vi "Controls-Loop.vi"(7 "JSON cmd queue":refnum<queue>, 8 "error in":errorcluster, 9 "Control Data Notifier":refnum<notifier>, 11 "Message Queues":T1) -> (0 "error out":errorcluster)   [LabVIEW 2024]
uses:
  support/Message Queue/All Message Queues.ctl
  support/Message Queue/Message Cluster.ctl
  support/Control/Control Data Constant.ctl
  support/Control/StreamCluster_TypeDef.ctl
  <vilib>/ErrorRing/Error Ring.xnode
  support/Message Queue/Message Queue.lvlib
  Controls State.ctl
  support/Control/DAQmx Container.ctl
  Sequence/Sequence Structure.ctl
  support/Control/BBControl Parameters.ctl
  332b4253-326d-4d7b-9710-a01b345fab27.vi
  61c51413-b1d0-41cf-878e-839bc20d578b.vi
  c894b992-033a-4c8a-923e-e5ce24f73376.vi
  Globals.vi
  <vilib>/MediaMongrels Ltd/WebSockets/WebSockets/WebSocket Server/WebSocket Server.lvclass
  support/Control/wsControlStates.ctl
  <vilib>/JDP Science/JSONtext/JSONtext.lvlib
  a787d3b8-bd60-4c2f-a7c4-6a756d9c913a.vi
  81e338ed-8fff-406a-9241-f88d912df8f4.vi
  a40d114d-95b6-498c-b24b-cea1f821b3b0.vi
  f3c74be8-3d28-4f30-9817-3fb28c56d5a3.vi
panel:
  out "Loop-3 Iteration Clock (s) 2":dbl format="%10.8f"
  out "Loop-3 Iteration Counter 2":i32
  out "Loop-3 Iteration Counter":i32
  out "Loop-3 Iteration Clock (s)":dbl format="%10.8f"
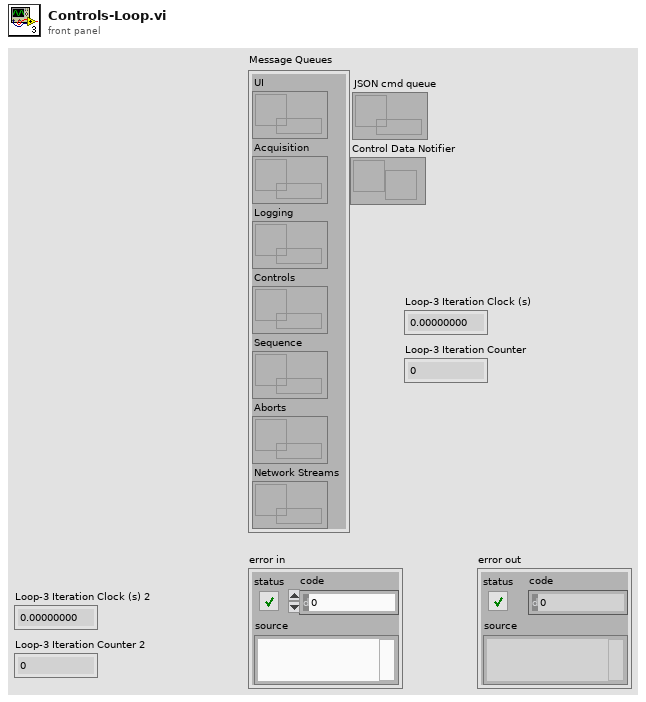
[diagram p1: front panel]
types:
  T1 = typedef "Message Queue.lvlib/All Message Queues.ctl" = cluster{"UI":refnum<queue>, "Acquisition":refnum<queue>, "Logging":refnum<queue>, "Controls":refnum<queue>, "Sequence":refnum<queue>, "Aborts":refnum<queue>, "Network Streams":refnum<queue>}
  T2 = typedef "wsControlStates.ctl" = enum16{"state_req", "state_update", "entrySequence", "control", "exitSequence"}
  T3 = cluster{"cmd set index":i32, "cmd subset index":i32, "cmd value":dbl, "t_ms":dbl, "refDes":string}
  T4 = typedef "Control Data Constant.ctl" = cluster{"Time (utc)":ext, "Data Out":cluster{"DO":bool[], "Module Number":string}[]}
  T5 = typedef "StreamCluster_TypeDef.ctl" = cluster{"DAQ":cluster{"ManagmentRate_Hz":i32, "StreamRate_Hz":i32, "StreamRate_ms":i32, "ManagmentRate_ms":i32, "refDesArray":cluster{"refDes-s":string[], "Module Number":string}[]}, "Modules":cluster{"Slot ID":i32, "Model Number":string, "Sample Rate s/S (Hz)":dbl, "Sensors":cluster{"refDes":string, "serialNumber":string, "modelNumber":string, "units":string, "balance":dbl, "sensitivity":dbl, "type":string, "inputTerminalConfiguration":string, "channelNumber":string, "taskName":string, "bridgeConfiguration":string, "excitationVoltage":dbl, "voltageExcitationSource":string, "nominalBridgeResistance":dbl, "firstElectricalValue":dbl, "secondElectricalValue":dbl, "firstPhysicalValue":dbl, "secondPhysicalValue":dbl, "electricalUnits":string}[]}[]}
  T6 = cluster{"refDes-s":string[], "Module Number":string}[]
  T7 = typedef "Controls State.ctl" = enum16{"Idle", "Control", "Sequencing", "Abort"}
  T8 = typedef "BBControl Parameters.ctl" = cluster{"Sequence Delay (s)":dbl, "Sequence Duration (s)":dbl, "BBControl Criteria":cluster{"Channel Name":i32, "Comparison":u16, "Set":dbl, "Enabled":bool, "Valve Name":i32, "Upper":dbl, "Lower":dbl}[]}
  T9 = typedef "DAQmx Container.ctl" = cluster{"DAQmx Analog In":refnum<k21>, "DAQmx Digital In":refnum<k21>, "DAQmx Digital Out":refnum<k21>, "DAQmx Analog Out":refnum<k21>, "DAQmx 6343":refnum<k21>, "DAQmx IG-Sense":refnum<k21>, "DAQmx Thermo":refnum<k21>, "DAQmx Bridge":refnum<k21>, "DAQmx Trigger":refnum<k21>}
  T10 = typedef "Sequence Structure.ctl" = cluster{"Sequence Controller":cluster{"Time (s)":dbl, "Enabled":bool, "Valve":u16[]}[], "Sequence Delay":dbl, "Sequence Duration":dbl}
  T11 = typedef "LVDateTimeRec.ctl" = cluster{"fractional second":dbl, "second":i32, "minute":i32, "hour":i32, "day of month":i32, "month":i32, "year":i32, "day of week":i32, "day of year":i32, "DST":i32}
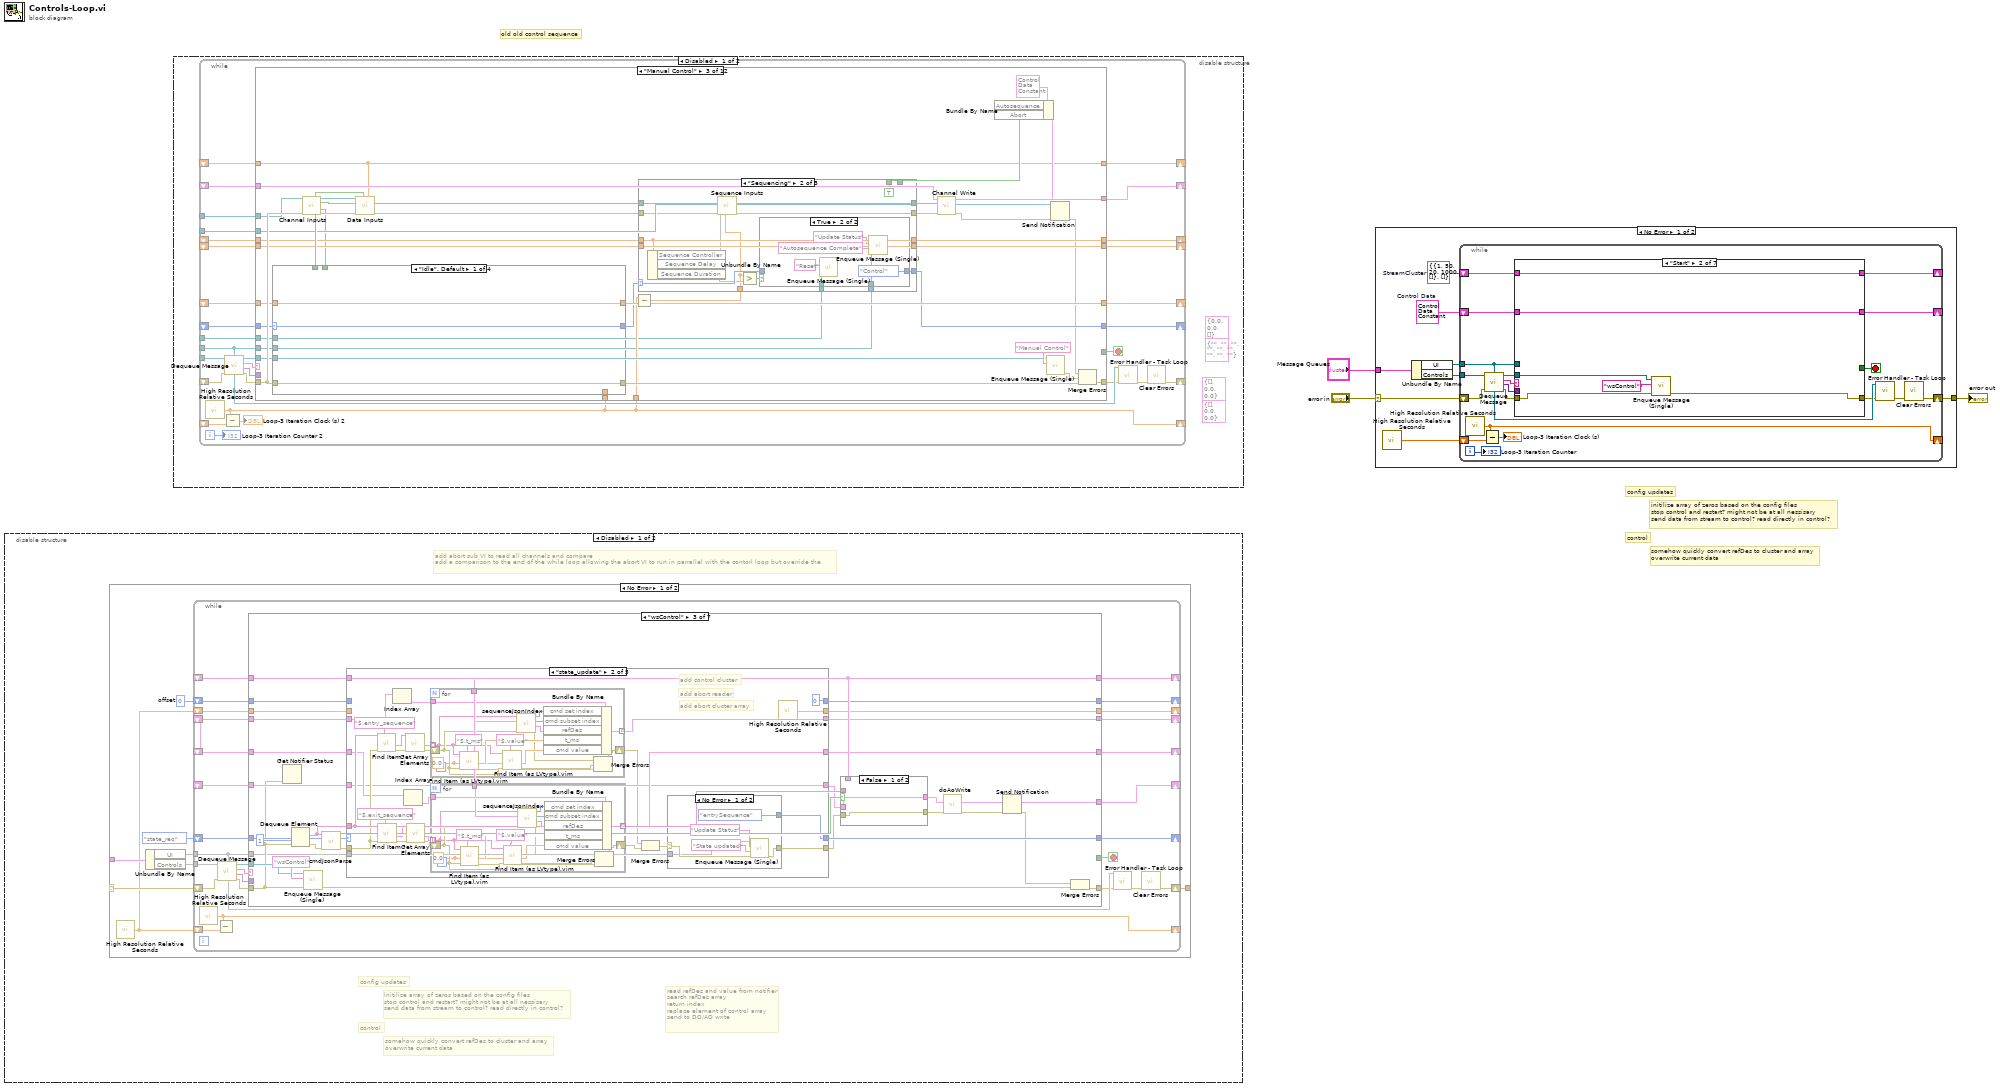
[diagram p0: block diagram]
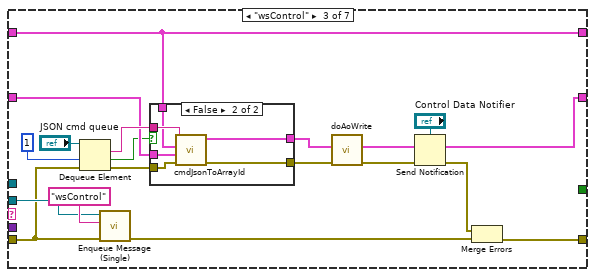
[diagram p3: hidden frame]
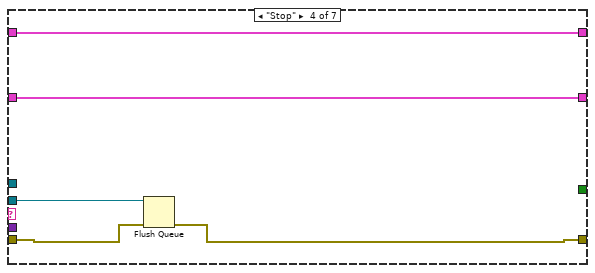
[diagram p5: hidden frame]
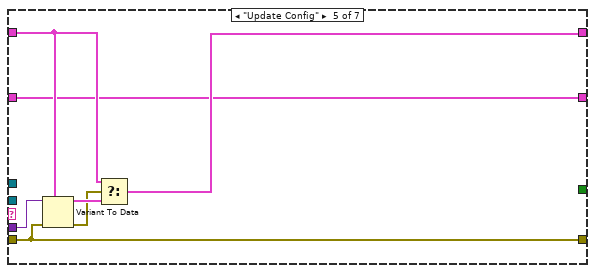
[diagram p6: hidden frame]
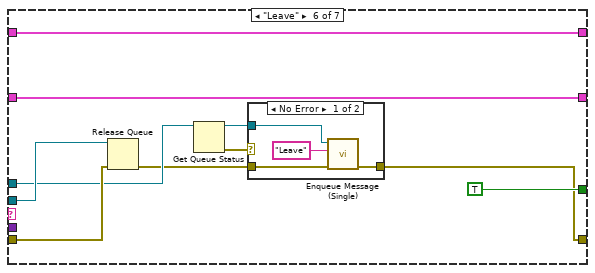
[diagram p7: hidden frame]
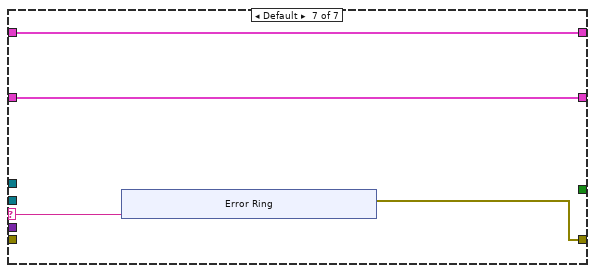
[diagram p9: hidden frame]
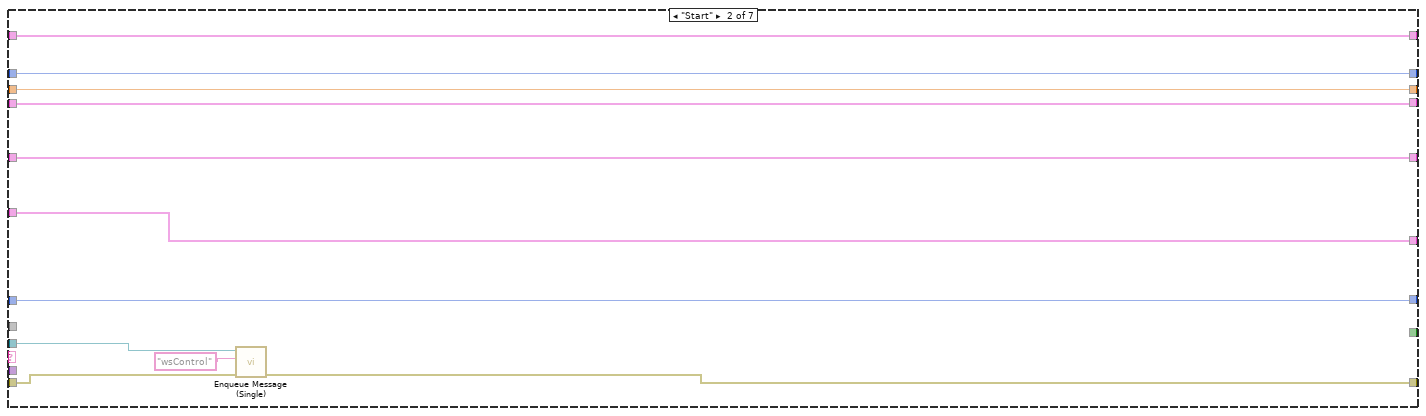
[diagram p12: hidden frame]
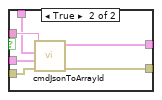
[diagram p13: hidden frame]
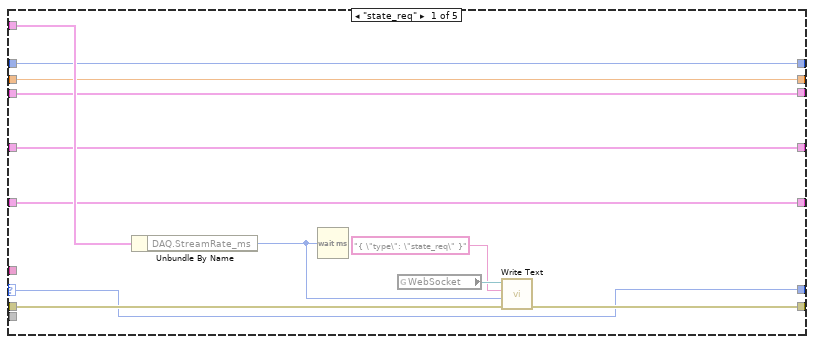
[diagram p14: hidden frame]
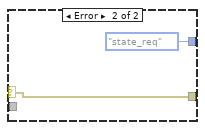
[diagram p15: hidden frame]
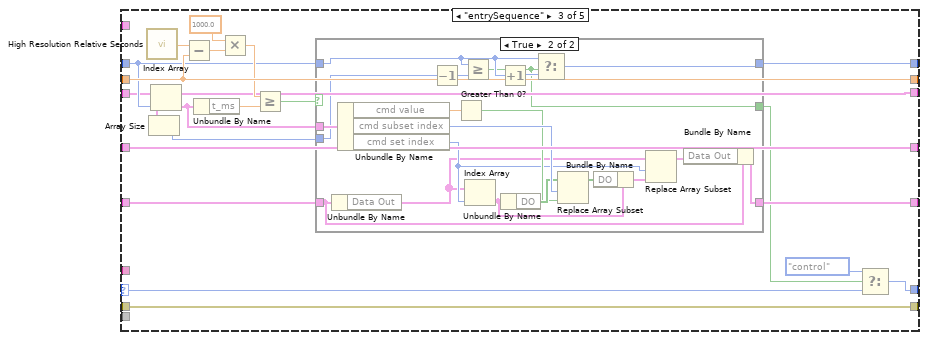
[diagram p16: hidden frame]
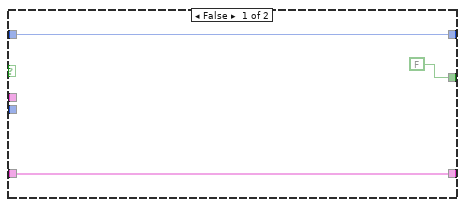
[diagram p17: hidden frame]
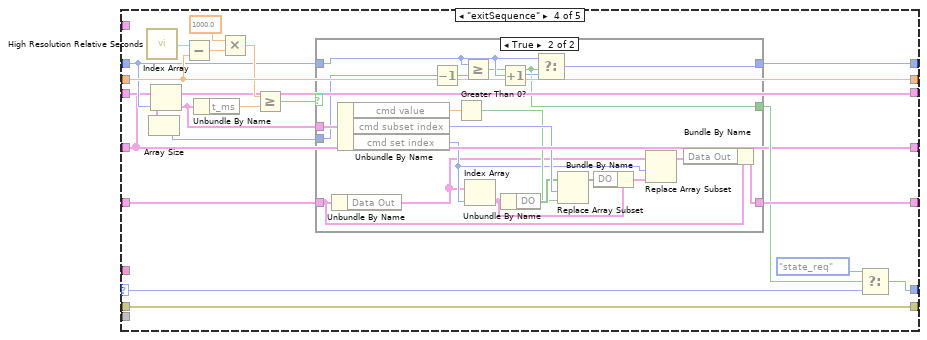
[diagram p18: hidden frame]
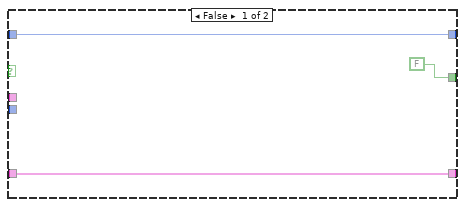
[diagram p19: hidden frame]
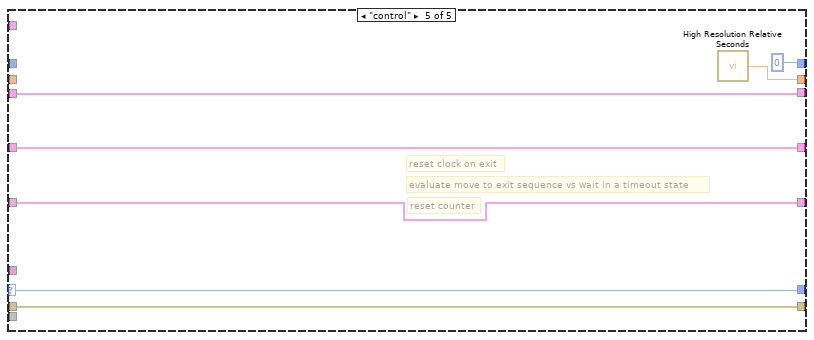
[diagram p20: hidden frame]
diagram:
  # "somehow quickly convert refDes to cluster and array\noverwrite current data"
  # "control"
  # "initilize array of zeros based on the config files \nstop control and restart? might not be at all nessisary\nsend data from stream to control? read directly in control?"
  # "config updates"
  # "old old control sequence"
  n1 = disable-structure shown="Disabled" {
    frame Disabled {
      # "add abort sub VI to read all channels and compare\nadd a comparison to the end of the while loop allowing the abort VI to run in parrallel with the contorl loop but override the"
      # "read refDes and value from notifier\nsearch refDes array\nreturn index\nreplace element of control array\nsend to DO/AO write"
      # "somehow quickly convert refDes to cluster and array\noverwrite current data"
      # "control"
      # "initilize array of zeros based on the config files \nstop control and restart? might not be at all nessisary\nsend data from stream to control? read directly in control?"
      # "config updates"
      n2 = case shown="No Error" w5 {
        selector: [w16 w347] -> w5
        tunnel: [w15 w347] -> _
        tunnel: [w14 _] -> w4
        frame No Error {
          w7 = 0  # offset
          n3 = call <vilib>:"High Resolution Relative Seconds.vi"() -> ("relative seconds"=w6:dbl)
          n4 = Unbundle By Name(w14) -> ("UI"=w13, "Controls"=w12)
          n5 = while {
            shift-right: [w32] -> w15
            shift-left: w16 -> [w42]
            tunnel: w13 -> [w36]
            tunnel: w12 -> [w43]
            shift-right: [w31] -> _
            shift-left: w6 -> [w35]
            shift-right: [w28] -> _
            shift-left: [w30] -> w11
            shift-right: [w27] -> _
            shift-left: [w29] -> w10
            shift-right: [w25] -> _
            shift-left: wsControlStates."state_req" -> [w26]
            shift-right: [w22] -> _
            shift-left: [w23] -> w8
            shift-right: [w21] -> _
            shift-left: w8 -> [w24]
            shift-right: [w17] -> _
            shift-left: w7 -> [w20]
            shift-right: [w18] -> _
            shift-left: w6 -> [w19]
            i -> [w34]
            stop <- w37 stop-if-true
            n6 = call <vilib>:"High Resolution Relative Seconds.vi"() -> ("relative seconds"=w31:dbl)
            n7 = Subtract(x=w31, y=w35) -> ()  [unwired: 1 out]
            n8 = call "Dequeue Message.vi"("error in (no error)"=w42, "Message Queue"=w43) -> ("error out"=w41:errorcluster, "Message Data"=w39:variant, "Message"=w38:string, "dup Message Queue"=w40:refnum<queue>)  [unwired: 6 in]
            n9 = case shown="\"wsControl\"" w38 {
              selector: w38 -> [_ _ _ _ _ _ w340]
              tunnel: [w52 w61 w94 w284 w302 w324 w341] -> w33
              tunnel: w41 -> [w52 w62 w77 w285 w302 w326 _]
              tunnel: w40 -> [_ w63 w92 w283 _ w327 _]
              tunnel: w39 -> [_ _ _ _ w303 _ _]
              tunnel: [_ _ _ _ _ TRUE _] -> w37
              tunnel: w36 -> [_ _ w71 _ _ w323 _]
              tunnel: w30 -> [w51 w60 w85 w282 w294 w318 w338]
              tunnel: w29 -> [w50 w59 w88 w281 w293 w319 w339]
              tunnel: [w51 w60 w82 w282 w292 w318 w338] -> w28
              tunnel: [w50 w59 w88 w281 w291 w319 w339] -> w27
              tunnel: w26 -> [w49 w57 w78 _ w290 w317 w337]
              tunnel: [w49 w57 w87 wsControlStates."state_req" ("controlStates") w290 w317 w337] -> w25
              tunnel: w24 -> [w48 w53 w73 w279 w286 w313 w333]
              tunnel: w23 -> [w47 w54 w72 w278 w287 w314 w334]
              tunnel: [w47 w54 w70 w278 w287 w314 w334] -> w22
              tunnel: [w48 w53 w69 w279 w286 w313 w333] -> w21
              tunnel: w20 -> [w45 w56 w67 w276 w289 w316 w336]
              tunnel: w19 -> [w46 w55 w66 w277 w288 w315 w335]
              tunnel: [w46 w55 w65 w277 w288 w315 w335] -> w18
              tunnel: [w45 w56 w64 w276 w289 w316 w336] -> w17
              frame "Initialize" {
              }
              frame "Start" {
                n10 = call "Enqueue Message (Single).vi"("error in (no error)"=w62, "Message"="wsControl", "Message Queue"=w63) -> ("error out"=w61:errorcluster)  [unwired: 7 in, 1 out]
              }
              frame "wsControl" {
                n11 = Get Notifier Status(error in (no error)=w77) -> ()  [unwired: 1 in, 5 out]
                n12 = Dequeue Element(timeout in ms (-1)=1, error in (no error)=w77) -> (element=w74:string, error out=w90:errorcluster)  [unwired: 1 in, 2 out]
                n13 = call "Enqueue Message (Single).vi"("error in (no error)"=w77, "Message"="wsControl", "Message Queue"=w92) -> ("error out"=w80:errorcluster)  [unwired: 7 in, 1 out]
                n14 = call "cmdJsonParse.vi"("error in"=w90, "controlStates"=w78, "cmdJson"=w74) -> ("error out"=w75:errorcluster, "controlStates"=w76:T2, "cmd"=w89:bool)  [unwired: 6 in]
                n15 = case shown="\"state_update\"" w76 {
                  selector: w76 -> [w105 _ w189 w232 w270]
                  tunnel: [w113 w117 w204 w246 w269] -> w84
                  tunnel: w75 -> [w112 w135 w204 w246 w269]
                  tunnel: w88 -> [w111 w125 _ _ _]
                  tunnel: [w105 w118 w186 w229 w270] -> w87
                  tunnel: w85 -> [w108 w123 w195 w238 w271]
                  tunnel: [w108 w123 w194 w237 w271] -> w68
                  tunnel: w74 -> [_ w136 _ _ _]
                  tunnel: w73 -> [w106 w126 w203 w227 w272]
                  tunnel: w72 -> [w107 w133 w185 w228 w273]
                  tunnel: w71 -> [_ w119 _ _ _]
                  tunnel: [w107 w131 w185 w228 w273] -> w70
                  tunnel: [w106 w124 w203 w227 w272] -> w69
                  tunnel: w67 -> [w104 _ w192 w235 _]
                  tunnel: w66 -> [w103 _ w201 w244 _]
                  tunnel: [w103 w116 w201 w244 w274] -> w65
                  tunnel: [w104 0 ("offset") w191 w234 0 ("offset")] -> w64
                  frame "state_req" {
                    n16 = Unbundle By Name(w111) -> ("DAQ.StreamRate_ms"=w109:i32)
                    n17 = Wait (ms)(milliseconds to wait=w109) -> ()  [unwired: 1 out]
                    n18 = global read "Globals.vi" "WebSocket"() -> (w114:refnum<class "WebSocket Server.lvclass">)
                    n19 = call-dynamic "Write Text.vi"("error in (no error)"=w112, "timeout ms (5000)"=w109, "String Data"="{ \"type\": \"state_req\" }", "WebSocket in"=w114) -> ("error out"=w113:errorcluster)  [unwired: 6 in, 1 out]
                  }
                  frame "state_update" {
                    # "add control cluster"
                    # "add abort cluster array"
                    # "add abort reader"
                    n20 = call <vilib>:"Find Item.vi"("$Path or Item Name"="$.entry_sequence", "error in (no error)"=w135, "JSON"=w136) -> ("error out"=w139:errorcluster, "<JSON>"=w138:string)  [unwired: 5 in, 2 out]
                    n21 = call <vilib>:"Find Item.vi"("$Path or Item Name"="$.exit_sequence", "error in (no error)"=w135, "JSON"=w136) -> ("error out"=w142:errorcluster, "<JSON>"=w141:string)  [unwired: 5 in, 2 out]
                    n22 = Index Array(array=w133) -> (element=w132:T3)  [unwired: 1 in]
                    n23 = Index Array(array=w126) -> (element=w127:T3)  [unwired: 1 in]
                    n24 = call <vilib>:"Get Array Elements.vi"("error in (no error)"=w139, "JSON"=w138) -> ("error out"=w130:errorcluster, "<JSON>"=w134:string[])  [unwired: 7 in, 1 out]
                    n25 = call <vilib>:"Get Array Elements.vi"("error in (no error)"=w142, "JSON"=w141) -> ("error out"=w128:errorcluster, "<JSON>"=w129:string[])  [unwired: 7 in, 1 out]
                    n26 = for {
                      tunnel: w134 -> [w172] mode=indexing
                      tunnel: w132 -> [w184]
                      tunnel: [w181] -> w131 mode=indexing
                      shift-right: [w168] -> w121
                      shift-left: w130 -> [w175]
                      tunnel: w125 -> [w180]
                      w174 = 0.0
                      n27 = call "Find Item (as LVtype).vim"("$Path or Item Name"="$.t_ms", "error in (no error)"=w175, "Data Type and Default Value"=w174, "JSON"=w172) -> ("error out"=w171:errorcluster, "Data"=w177:dbl)  [unwired: 4 in, 2 out]
                      n28 = call "Find Item (as LVtype).vim"("$Path or Item Name"="$.value", "error in (no error)"=w175, "Data Type and Default Value"=w174, "JSON"=w172) -> ("error out"=w170:errorcluster, "Data"=w173:dbl)  [unwired: 4 in, 2 out]
                      n29 = call "sequenceJsonIndex.vi"("error in"=w175, "StreamCluster"=w180, "JSON in"=w172) -> ("error out"=w169:errorcluster, "refDes"=w179:string, "cmd subset index"=w182:i32, "cmd set index"=w183:i32)  [unwired: 5 in]
                      n30 = Bundle By Name(cluster=w184, "cmd set index"=w183, "cmd subset index"=w182, "refDes"=w179, "t_ms"=w177, "cmd value"=w173) -> (w181:T3)
                      n31 = Merge Errors(w169, w170, w171) -> (w168:errorcluster)
                    }
                    n32 = for {
                      tunnel: w129 -> [w155] mode=indexing
                      tunnel: w127 -> [w167]
                      tunnel: [w164] -> w124 mode=indexing
                      shift-right: [w151] -> w122
                      shift-left: w128 -> [w158]
                      tunnel: w125 -> [w163]
                      w157 = 0.0
                      n33 = call "Find Item (as LVtype).vim"("$Path or Item Name"="$.t_ms", "error in (no error)"=w158, "Data Type and Default Value"=w157, "JSON"=w155) -> ("error out"=w154:errorcluster, "Data"=w160:dbl)  [unwired: 4 in, 2 out]
                      n34 = call "Find Item (as LVtype).vim"("$Path or Item Name"="$.value", "error in (no error)"=w158, "Data Type and Default Value"=w157, "JSON"=w155) -> ("error out"=w153:errorcluster, "Data"=w156:dbl)  [unwired: 4 in, 2 out]
                      n35 = call "sequenceJsonIndex.vi"("error in"=w158, "StreamCluster"=w163, "JSON in"=w155) -> ("error out"=w152:errorcluster, "refDes"=w162:string, "cmd subset index"=w165:i32, "cmd set index"=w166:i32)  [unwired: 5 in]
                      n36 = Bundle By Name(cluster=w167, "cmd set index"=w166, "cmd subset index"=w165, "refDes"=w162, "t_ms"=w160, "cmd value"=w156) -> (w164:T3)
                      n37 = Merge Errors(w152, w153, w154) -> (w151:errorcluster)
                    }
                    n38 = Merge Errors(w121, w122) -> (w120:errorcluster)
                    n39 = case shown="No Error" w120 {
                      selector: w120 -> [w147 w149]
                      tunnel: w119 -> [w145 _]
                      tunnel: [wsControlStates."entrySequence" wsControlStates."state_req"] -> w118
                      tunnel: [w143 w149] -> w117
                      frame No Error {
                        n40 = call "Enqueue Message (Single).vi"("error in (no error)"=w147, "Message Data"="State updated", "Message"="Update Status", "Message Queue"=w145) -> ("error out"=w143:errorcluster)  [unwired: 6 in, 1 out]
                      }
                      frame Error {
                      }
                    }
                    n41 = call <vilib>:"High Resolution Relative Seconds.vi"() -> ("relative seconds"=w116:dbl)
                  }
                  frame "entrySequence" {
                    n42 = call <vilib>:"High Resolution Relative Seconds.vi"() -> ("relative seconds"=w202:dbl)
                    n43 = Array Size(array=w185) -> (size(s)=w190:i32)
                    n44 = Index Array(array=w185, index=w192) -> (element=w193:T3)
                    n45 = Subtract(x=w202, y=w201) -> (x-y=w200:dbl)
                    n46 = Unbundle By Name(w193) -> ("t_ms"=w198:dbl)
                    n47 = Multiply(x=1000.0, y=w200) -> (x*y=w197:dbl)
                    n48 = Greater Or Equal?(x=w197, y=w198) -> (x >= y?=w196:bool)
                    n49 = case shown="True" w196 {
                      tunnel: w195 -> [w207 w212]
                      tunnel: [w207 w211] -> w194
                      tunnel: w193 -> [_ w223]
                      tunnel: w192 -> [w206 w224]
                      tunnel: [w206 w225] -> w191
                      tunnel: w190 -> [_ w209]
                      tunnel: [FALSE w210] -> w188
                      frame False {
                      }
                      frame True {
                        n50 = Unbundle By Name(w212) -> ("Data Out"=w214:cluster{"DO":bool[], "Module Number":string}[])
                        n51 = Unbundle By Name(w223) -> ("cmd value"=w222:dbl, "cmd subset index"=w221:i32, "cmd set index"=w215:i32)
                        n52 = Decrement(x=w209) -> (x-1=w208:i32)
                        n53 = Greater Than 0?(x=w222) -> (x > 0?=w219:bool)
                        n54 = Greater Or Equal?(x=w224, y=w208) -> (x >= y?=w210:bool)
                        n55 = Index Array(array=w214, index=w215) -> (element=w218:cluster{"DO":bool[], "Module Number":string})
                        n56 = Increment(x=w224) -> (x+1=w226:i32)
                        n57 = Unbundle By Name(w218) -> ("DO"=w220:bool[])
                        n58 = Select(t=w224, s=w210, f=w226) -> (s? t:f=w225:i32)
                        n59 = Replace Array Subset(array=w220, new element=w219, index=w221) -> (w217:bool[])
                        n60 = Bundle By Name(cluster=w218, "DO"=w217) -> (w216:cluster{"DO":bool[], "Module Number":string})
                        n61 = Replace Array Subset(array=w214, new element=w216, index=w215) -> (w213:cluster{"DO":bool[], "Module Number":string}[])
                        n62 = Bundle By Name(cluster=w212, "Data Out"=w213) -> (w211:T4)
                      }
                    }
                    n63 = Select(t=wsControlStates."control", s=w188, f=w189) -> (s? t:f=w186:T2)
                  }
                  frame "exitSequence" {
                    n64 = call <vilib>:"High Resolution Relative Seconds.vi"() -> ("relative seconds"=w245:dbl)
                    n65 = Array Size(array=w227) -> (size(s)=w233:i32)
                    n66 = Index Array(array=w227, index=w235) -> (element=w236:T3)
                    n67 = Subtract(x=w245, y=w244) -> (x-y=w243:dbl)
                    n68 = Unbundle By Name(w236) -> ("t_ms"=w241:dbl)
                    n69 = Multiply(x=1000.0, y=w243) -> (x*y=w240:dbl)
                    n70 = Greater Or Equal?(x=w240, y=w241) -> (x >= y?=w239:bool)
                    n71 = case shown="True" w239 {
                      tunnel: w238 -> [w249 w254]
                      tunnel: [w249 w253] -> w237
                      tunnel: w236 -> [_ w265]
                      tunnel: w235 -> [w248 w266]
                      tunnel: [w248 w267] -> w234
                      tunnel: w233 -> [_ w251]
                      tunnel: [FALSE w252] -> w231
                      frame False {
                      }
                      frame True {
                        n72 = Unbundle By Name(w254) -> ("Data Out"=w256:cluster{"DO":bool[], "Module Number":string}[])
                        n73 = Unbundle By Name(w265) -> ("cmd value"=w264:dbl, "cmd subset index"=w263:i32, "cmd set index"=w257:i32)
                        n74 = Decrement(x=w251) -> (x-1=w250:i32)
                        n75 = Greater Than 0?(x=w264) -> (x > 0?=w261:bool)
                        n76 = Greater Or Equal?(x=w266, y=w250) -> (x >= y?=w252:bool)
                        n77 = Index Array(array=w256, index=w257) -> (element=w260:cluster{"DO":bool[], "Module Number":string})
                        n78 = Increment(x=w266) -> (x+1=w268:i32)
                        n79 = Unbundle By Name(w260) -> ("DO"=w262:bool[])
                        n80 = Select(t=w266, s=w252, f=w268) -> (s? t:f=w267:i32)
                        n81 = Replace Array Subset(array=w262, new element=w261, index=w263) -> (w259:bool[])
                        n82 = Bundle By Name(cluster=w260, "DO"=w259) -> (w258:cluster{"DO":bool[], "Module Number":string})
                        n83 = Replace Array Subset(array=w256, new element=w258, index=w257) -> (w255:cluster{"DO":bool[], "Module Number":string}[])
                        n84 = Bundle By Name(cluster=w254, "Data Out"=w255) -> (w253:T4)
                      }
                    }
                    n85 = Select(t=wsControlStates."state_req", s=w231, f=w232) -> (s? t:f=w229:T2)
                  }
                  frame "control" {
                    # "reset counter"
                    # "evaluate move to exit sequence vs wait in a timeout state"
                    # "reset clock on exit"
                    n86 = call <vilib>:"High Resolution Relative Seconds.vi"() -> ("relative seconds"=w274:dbl)
                  }
                }
                n87 = case shown="False" w89 {
                  tunnel: [w95 w102] -> w86
                  tunnel: w74 -> [_ w101]
                  tunnel: w88 -> [_ w100]
                  tunnel: w68 -> [w96 w99]
                  tunnel: [w96 w98] -> w83
                  tunnel: w84 -> [w95 w97]
                  frame False {
                  }
                  frame True {
                    n88 = call "cmdJsonToArrayId.vi"("error in"=w97, "Control Data"=w99, "StreamCluster"=w100, "JSON in"=w101) -> ("error out"=w102:errorcluster, "Control Data"=w98:T4)  [unwired: 6 in]
                  }
                }
                n89 = call "doAoWrite.vi"("error in"=w86, "Control Data"=w83) -> ("error out"=w91:errorcluster, "Control Data"=w82:T4)  [unwired: 7 in, 1 out]
                n90 = Send Notification(notification=w82, error in (no error)=w91) -> (error out=w81:errorcluster)  [unwired: 1 in, 1 out]
                n91 = Merge Errors(w81, w80) -> (w94:errorcluster)
              }
              frame "Stop" {
                n92 = Flush Queue(queue=w283, error in (no error)=w285) -> (error out=w284:errorcluster)  [unwired: 2 out]
              }
              frame "Update Config" {
                n93 = Variant To Data(error in=w302, type=w293, Variant=w303) -> (data=w304:T5, error out=w301:errorcluster)
                n94 = Select(t=w293, s=w301, f=w304) -> (s? t:f=w291:T5)
                n95 = Unbundle By Name(w291) -> ("DAQ.refDesArray"=w295:T6)
                n96 = Array Size(array=w295) -> (size(s)=w298:i32)
                n97 = Unbundle By Name(w294) -> ("Data Out"=w297:cluster{"DO":bool[], "Module Number":string}[])
                n98 = Index Array(array=w297) -> (element=w296:cluster{"DO":bool[], "Module Number":string})  [unwired: 1 in]
                n99 = for {
                  N: w298 -> [_]
                  tunnel: w295 -> [w307] mode=indexing
                  tunnel: w296 -> [w310]
                  tunnel: [w308] -> w300 mode=indexing
                  n100 = Unbundle(w307) -> ("refDes-s"=w306:string[], "Module Number"=w305:string)
                  n101 = Array Size(array=w306) -> (size(s)=w311:i32)
                  n102 = Initialize Array(FALSE, w311) -> (w309:bool[])
                  n103 = Bundle By Name(cluster=w310, "DO"=w309, "Module Number"=w305) -> (w308:cluster{"DO":bool[], "Module Number":string})
                }
                n104 = Bundle By Name(cluster=w294, "Data Out"=w300) -> (w299:T4)
                n105 = Select(t=w294, s=w301, f=w299) -> (s? t:f=w292:T4)
              }
              frame "Leave" {
                n106 = Release Queue(queue=w327, error in (no error)=w326) -> (error out=w321:errorcluster)  [unwired: 1 in, 2 out]
                n107 = Get Queue Status(queue=w323) -> (queue out=w322:refnum<queue>, error out=w320:errorcluster)  [unwired: 2 in, 6 out]
                n108 = case shown="No Error" w320 {
                  tunnel: [w330 w332] -> w324
                  tunnel: w322 -> [w329 _]
                  tunnel: w321 -> [w328 w332]
                  frame No Error {
                    n109 = call "Enqueue Message (Single).vi"("error in (no error)"=w328, "Message"="Leave", "Message Queue"=w329) -> ("error out"=w330:errorcluster)  [unwired: 7 in, 1 out]
                  }
                  frame Error {
                  }
                }
              }
              frame Default {
                n110 = xnode "Error Ring"("parameter 0"=w340) -> ("error out"=w341:errorcluster)
              }
            }
            n111 = call "Error Handler - Task Loop.vi"("error in (no error)"=w33, "Message Queue"=w36) -> ("dup error in"=w44:errorcluster)  [unwired: 8 in, 1 out]
            n112 = call <vilib>:"Clear Errors.vi"("error in (no error)"=w44) -> ("error out"=w32:errorcluster)  [unwired: 5 in, 1 out]
          }
        }
        frame Error {
        }
      }
    }
    frame Enabled {
    }
  }
  n113 = disable-structure shown="Disabled" {
    frame Disabled {
      (unwired) T8 {"Sequence Delay (s)"=0.0, "Sequence Duration (s)"=0.0, "BBControl Criteria"=[]} ("BBControl Parameters")
      (unwired) T9 {"DAQmx Analog In"="", "DAQmx Digital In"="", "DAQmx Digital Out"="", "DAQmx Analog Out"="", "DAQmx 6343"="", "DAQmx IG-Sense"="", "DAQmx Thermo"="", "DAQmx Bridge"="", "DAQmx Trigger"=""} ("DAQmx Container")
      (unwired) T10 {"Sequence Controller"=[], "Sequence Delay"=0.0, "Sequence Duration"=0.0} ("Sequence Conditions")
      (unwired) T10 {"Sequence Controller"=[], "Sequence Delay"=0.0, "Sequence Duration"=0.0} ("Sequence Conditions")
      n114 = while {
        shift-right: [w350] -> _
        shift-left: _ -> [w375]
        tunnel: _ -> [w367]
        tunnel: _ -> [w376]
        shift-right: [w369] -> _
        shift-left: _ -> [w370]
        shift-right: [w357] -> _
        shift-left: _ -> [w365]
        tunnel: _ -> [w362]
        shift-right: [w360] -> _
        shift-left: _ -> [w361]
        tunnel: _ -> [w359]
        tunnel: _ -> [w358]
        shift-right: [w356] -> _
        shift-left: _ -> [w355]
        shift-right: [w353] -> _
        shift-left: _ -> [w354]
        shift-right: [w351] -> _
        shift-left: _ -> [w352]
        shift-right: [w348] -> _
        shift-left: _ -> [w349]
        i -> [w364]
        stop <- w368 stop-if-true
        n115 = call <vilib>:"High Resolution Relative Seconds.vi"() -> ("relative seconds"=w357:dbl)
        n116 = Subtract(x=w357, y=w365) -> (x-y=→"Loop-3 Iteration Clock (s) 2":dbl)
        n117 = call "Dequeue Message.vi"("error in (no error)"=w375, "Message Queue"=w376) -> ("error out"=w374:errorcluster, "Message Data"=w372:variant, "Message"=w371:string, "dup Message Queue"=w373:refnum<queue>)  [unwired: 6 in]
        n118 = case shown="\"Manual Control\"" w371 {
          selector: w371 -> [_ _ _ _ _ _ _ _ _ _ _ w686]
          tunnel: [w384 w390 w439 w590 w597 w604 w620 w630 w643 w654 w670 w687] -> w363
          tunnel: w374 -> [w384 w391 w442 w570 w597 w605 w622 w630 w643 w654 w673 _]
          tunnel: w373 -> [_ w392 w434 w586 _ w603 w621 _ _ _ w674 _]
          tunnel: w372 -> [_ _ _ _ _ _ w624 w636 w647 w658 _ _]
          tunnel: w370 -> [w383 w394 w440 w574 _ w607 w623 w635 w646 w657 w671 w685]
          tunnel: [w383 w393 w418 w574 Controls_State."Abort" ("Controls State") w606 w623 w635 w646 w657 w671 w685] -> w369
          tunnel: [w382 w389 w438 w589 w593 w602 w625 w631 w644 w655 w665 w684] -> w360
          tunnel: [_ _ _ _ _ _ _ _ _ _ TRUE _] -> w368
          tunnel: w367 -> [_ _ w413 _ _ _ _ _ _ _ w669 _]
          tunnel: w362 -> [_ _ w436 _ _ _ _ _ _ _ _ _]
          tunnel: w361 -> [w382 w389 w437 w588 w593 w602 w618 w631 w644 w655 w665 w684]
          tunnel: w359 -> [_ _ w406 _ _ _ _ _ _ _ _ _]
          tunnel: w358 -> [_ _ w410 w582 _ _ _ _ _ _ _ _]
          tunnel: w357 -> [_ _ w432 _ w594 _ _ _ _ _ _ _]
          tunnel: w357 -> [_ _ w429 _ _ _ _ _ _ _ _ _]
          tunnel: [w381 w388 w430 w573 w594 w601 w617 w634 w645 w656 w664 w683] -> w356
          tunnel: w355 -> [w381 w388 w431 w573 _ w601 w617 w634 w645 w656 w664 w683]
          tunnel: w354 -> [w380 w387 w416 w571 w595 w600 w616 w633 w640 w653 w663 w682]
          tunnel: [w380 w387 w415 w571 w595 w600 w616 w632 w640 w653 w663 w682] -> w353
          tunnel: w352 -> [w379 w386 w417 w572 w596 w599 w615 w629 w642 w652 w662 w681]
          tunnel: [w379 w386 w414 w572 w596 w599 w615 w629 w641 w652 w662 w681] -> w351
          tunnel: w349 -> [w378 w385 w402 w580 w591 w598 w614 w628 w639 w651 w661 w680]
          tunnel: [w378 w385 w402 w580 w591 w598 w614 w628 w639 w650 w661 w680] -> w348
          frame "Initialize" {
          }
          frame "Start" {
            n119 = case shown="\"Idle\", Default" w394 {
              selector: w394 -> [_ w401]
              tunnel: [Controls_State."Control" ("Controls State") w401] -> w393
              tunnel: w392 -> [w398 _]
              tunnel: w391 -> [w396 w400]
              tunnel: [w395 w400] -> w390
              frame "Idle", Default {
                n120 = call "Enqueue Message (Single).vi"("error in (no error)"=w396, "Message"="wsControl", "Message Queue"=w398) -> ("error out"=w395:errorcluster)  [unwired: 7 in, 1 out]
              }
              frame "Control" {
              }
            }
          }
          frame "Manual Control" {
            n121 = call "Channel Inputs.vi"("Data Notifier"=w436, "error in"=w442) -> ("BangBang\nArm out"=w403:bool, "Data Notifier out"=w426:refnum<notifier>, "Actuation Array"=w425:bool[], "Auto-sequence"=w407:bool, "Abort"=w428:bool, "error out"=w427:errorcluster)  [unwired: 8 in]
            n122 = case shown="\"Idle\", Default" w440 {
              selector: w440 -> [w492 w498 w525 w552]
              tunnel: w434 -> [_ w500 w527 w554]
              tunnel: w442 -> [w491 w499 w526 w553]
              tunnel: [w491 w503 w529 w557] -> w441
              tunnel: [w492 w504 w530 w558] -> w424
              tunnel: w413 -> [_ w501 w528 w555]
              tunnel: w406 -> [_ w502 w520 w556]
              tunnel: w407 -> [_ w494 _ w548]
              tunnel: w428 -> [_ _ w524 w545]
              tunnel: w432 -> [_ w497 w523 w551]
              tunnel: [w490 w496 w522 w550] -> w430
              tunnel: w431 -> [w490 w495 w521 w549]
              frame "Idle", Default {
              }
              frame "Control" {
                n123 = call "RisingEdgeDetector.vim"("Data"=w494) -> ("Edge?"=w493:bool)  [unwired: 4 in]
                n124 = case shown="True" w493 {
                  tunnel: [w507 Controls_State."Sequencing" ("Controls State")] -> w504
                  tunnel: w502 -> [_ w518]
                  tunnel: w499 -> [w506 w516]
                  tunnel: [w506 w513] -> w503
                  tunnel: w501 -> [_ w510]
                  tunnel: w500 -> [_ _]
                  tunnel: w498 -> [w507 _]
                  tunnel: [w505 w512] -> w496
                  tunnel: w497 -> [_ w512]
                  tunnel: w495 -> [w505 _]
                  frame False {
                  }
                  frame True {
                    n125 = call "Enqueue Message (Single).vi"("error in (no error)"=w516, "Message"="Start", "Message Queue"=w518) -> ("error out"=w508:errorcluster)  [unwired: 7 in, 1 out]
                    n126 = call "Enqueue Message (Single).vi"("error in (no error)"=w508, "Message"="Autosequence Start", "Message Queue"=w510) -> ("error out"=w509:errorcluster)  [unwired: 7 in, 1 out]
                    n127 = call "Enqueue Message (Single).vi"("error in (no error)"=w509, "Message Data"="Autosequence Started", "Message"="Update Status", "Message Queue"=w510) -> ("error out"=w513:errorcluster)  [unwired: 6 in, 1 out]
                  }
                }
              }
              frame "Sequencing" {
                n128 = case shown="True" w524 {
                  tunnel: [w533 Controls_State."Abort" ("Controls State")] -> w530
                  tunnel: w520 -> [_ w542]
                  tunnel: w526 -> [w532 w541]
                  tunnel: [w532 w537] -> w529
                  tunnel: w528 -> [_ w536]
                  tunnel: w527 -> [_ _]
                  tunnel: w525 -> [w533 _]
                  tunnel: w523 -> [_ w534]
                  tunnel: [w531 w534] -> w522
                  tunnel: w521 -> [w531 _]
                  frame False {
                  }
                  frame True {
                    n129 = call "Enqueue Message (Single).vi"("error in (no error)"=w541, "Message"="Reset", "Message Queue"=w542) -> ("error out"=w538:errorcluster)  [unwired: 7 in, 1 out]
                    n130 = call "Enqueue Message (Single).vi"("error in (no error)"=w538, "Message Data"="Manual Abort", "Message"="Update Status", "Message Queue"=w536) -> ("error out"=w537:errorcluster)  [unwired: 6 in, 1 out]
                  }
                }
              }
              frame "Abort" {
                n131 = call "FallingEdgeDetector.vim"("Data"=w545) -> ("Edge?"=w544:bool)  [unwired: 4 in]
                n132 = Not(x=w548) -> (.not. x?=w546:bool)
                n133 = And(x=w546, y=w544) -> (x .and. y?=w547:bool)
                n134 = case shown="True" w547 {
                  tunnel: [w561 Controls_State."Control" ("Controls State")] -> w558
                  tunnel: w556 -> [_ _]
                  tunnel: w553 -> [w560 w562]
                  tunnel: [w560 w565] -> w557
                  tunnel: w555 -> [_ w564]
                  tunnel: w554 -> [_ _]
                  tunnel: w552 -> [w561 _]
                  tunnel: w551 -> [_ w563]
                  tunnel: [w559 w563] -> w550
                  tunnel: w549 -> [w559 _]
                  frame False {
                  }
                  frame True {
                    n135 = call "Enqueue Message (Single).vi"("error in (no error)"=w562, "Message Data"="Manual Control", "Message"="Update Status", "Message Queue"=w564) -> ("error out"=w565:errorcluster)  [unwired: 6 in, 1 out]
                  }
                }
              }
            }
            n136 = call "Data Inputs.vi"("BBControl Parameters"=w402, "Arm"=w403, "error in"=w427, "Actuation Array in"=w425, "Data Notifier"=w426) -> ("error out"=w423:errorcluster, "Actuation Array out"=w421:bool[])  [unwired: 4 in, 1 out]
            n137 = Subtract(x=w429, y=w430) -> (x-y=w419:dbl)
            n138 = case shown="\"Sequencing\"" w424 {
              selector: w424 -> [w445 w461 w483]
              tunnel: w423 -> [w447 w456 w479]
              tunnel: [w447 w455 w478] -> w422
              tunnel: w421 -> [w446 w453 w476]
              tunnel: [w446 w452 w475] -> w420
              tunnel: w419 -> [_ w454 w477]
              tunnel: [w445 w460 w482] -> w418
              tunnel: w417 -> [w443 w459 w473]
              tunnel: w416 -> [w444 w458 w481]
              tunnel: [w444 w458 w481] -> w415
              tunnel: [w443 w459 w473] -> w414
              tunnel: w413 -> [_ w450 w472]
              tunnel: [_ TRUE _] -> w405
              tunnel: w406 -> [_ w448 _]
              tunnel: [_ _ TRUE] -> w404
              frame Default {
              }
              frame "Sequencing" {
                n139 = Unbundle By Name(w458) -> ("Sequence Controller"=w451, "Sequence Duration"=w457)  [unwired: 1 out]
                n140 = call "Sequence Inputs.vi"("Time In"=w454, "error in"=w456, "Actuation Array in"=w453, "Sequence"=w451) -> ("error out"=w455:errorcluster, "Actuation Array out"=w452:bool[])  [unwired: 6 in]
                n141 = Greater?(x=w454, y=w457) -> (0:w462:bool)
                n142 = case shown="True" w462 {
                  tunnel: w461 -> [w463 _]
                  tunnel: [w463 Controls_State."Control" ("Controls State")] -> w460
                  tunnel: w450 -> [_ w466]
                  tunnel: w448 -> [_ w464]
                  frame False {
                  }
                  frame True {
                    n143 = call "Enqueue Message (Single).vi"("Message"="Reset", "Message Queue"=w464) -> ()  [unwired: 8 in, 2 out]
                    n144 = call "Enqueue Message (Single).vi"("Message Data"="Autosequence Complete", "Message"="Update Status", "Message Queue"=w466) -> ()  [unwired: 7 in, 2 out]
                  }
                }
              }
              frame "Abort" {
                n145 = Unbundle By Name(w473) -> ("Sequence Controller"=w474, "Sequence Duration"=w480)  [unwired: 1 out]
                n146 = call "Sequence Inputs.vi"("Time In"=w477, "error in"=w479, "Actuation Array in"=w476, "Sequence"=w474) -> ("error out"=w478:errorcluster, "Actuation Array out"=w475:bool[])  [unwired: 6 in]
                n147 = Greater?(x=w477, y=w480) -> (0:w484:bool)
                n148 = call "RisingEdgeDetector.vim"("Data"=w484) -> ("Edge?"=w471:bool)  [unwired: 4 in]
                n149 = case shown="True" w471 {
                  tunnel: w483 -> [w485 w486]
                  tunnel: [w485 w486] -> w482
                  tunnel: w472 -> [_ w487]
                  frame False {
                  }
                  frame True {
                    n150 = call "Enqueue Message (Single).vi"("Message Data"="Abort Sequence Complete", "Message"="Update Status", "Message Queue"=w487) -> ()  [unwired: 7 in, 2 out]
                  }
                }
              }
            }
            n151 = call "Channel Write.vi"("error in"=w422, "Actuation Array"=w420, "DAQmx Container In"=w437) -> ("error out"=w412:errorcluster, "DAQmx Container Out"=w438:T9)  [unwired: 6 in, 1 out]
            n152 = Bundle By Name(cluster=T4 {"Time (utc)"=0.0, "Data Out"=[]} ("notification"), "Autosequence"=w405, "Abort"=w404) -> (w408:T4)
            n153 = call "Enqueue Message (Single).vi"("Message"="Manual Control", "Message Queue"=w434) -> ("error out"=w433:errorcluster)  [unwired: 8 in, 1 out]
            n154 = Send Notification(notification=w408, notifier=w410, error in (no error)=w412) -> (error out=w411:errorcluster)  [unwired: 1 out]
            n155 = Merge Errors(w411, w433, w441) -> (w439:errorcluster)
          }
          frame "wsControl" {
            n156 = Get Date/Time In Seconds() -> (seconds since 1Jan1904=w578:timestamp)
            n157 = Seconds To Date/Time(time stamp (now)=w578, to UTC (F)=TRUE) -> (date time rec=w579:T11)
            n158 = call "doAoWrite.vi"("error in"=w570, "DAQmx Container In"=w588) -> ("error out"=w584:errorcluster, "Control Data"=w569:T4, "DAQmx Container Out"=w589:T9)  [unwired: 7 in]
            n159 = Date/Time To Seconds(2:w579) -> (0:w576:timestamp)  [unwired: 1 in]
            n160 = To Extended Precision Float(1:w576) -> (0:w575:ext)
            n161 = Bundle By Name(cluster=w569, "Time (utc)"=w575) -> (w581:T4)
            n162 = call "Enqueue Message (Single).vi"("Message"="wsControl", "Message Queue"=w586) -> ("error out"=w585:errorcluster)  [unwired: 8 in, 1 out]
            n163 = Send Notification(notification=w581, notifier=w582, error in (no error)=w584) -> (error out=w583:errorcluster)  [unwired: 1 out]
            n164 = Merge Errors(w583, w585, w570) -> (w590:errorcluster)
          }
          frame "Abort" {
          }
          frame "Stop" {
            n165 = case shown="\"Control\"" w607 {
              selector: w607 -> [w609 _]
              tunnel: [w609 Controls_State."Idle" ("Controls State")] -> w606
              tunnel: w605 -> [w608 w611]
              tunnel: [w608 w610] -> w604
              tunnel: w603 -> [_ w612]
              frame "Idle", Default {
              }
              frame "Control" {
                n166 = Flush Queue(queue=w612, error in (no error)=w611) -> (error out=w610:errorcluster)  [unwired: 2 out]
              }
            }
          }
          frame "Task Distribution" {
            n167 = Variant To Data(error in=w622, type=w618, Variant=w624) -> (data=w626:T9, error out=w627:errorcluster)
            n168 = Select(t=w618, s=w627, f=w626) -> (s? t:f=w625:T9)
            n169 = call "Enqueue Message (Single).vi"("error in (no error)"=w622, "Message"="Start", "Message Queue"=w621) -> ("error out"=w620:errorcluster)  [unwired: 7 in, 1 out]
          }
          frame "Update Sequence" {
            n170 = Variant To Data(error in=w630, type=w633, Variant=w636) -> (data=w637:dbl, error out=w638:errorcluster)
            n171 = Select(t=w633, s=w638, f=w637) -> (s? t:f=w632:dbl)
          }
          frame "Update AbortSequence" {
            n172 = Variant To Data(error in=w643, type=w642, Variant=w647) -> (data=w648:dbl, error out=w649:errorcluster)
            n173 = Select(t=w642, s=w649, f=w648) -> (s? t:f=w641:dbl)
          }
          frame "Update BBControl" {
            n174 = Variant To Data(error in=w654, type=w651, Variant=w658) -> (data=w659:dbl, error out=w660:errorcluster)
            n175 = Select(t=w651, s=w660, f=w659) -> (s? t:f=w650:dbl)
          }
          frame "Leave" {
            n176 = Release Queue(queue=w674, error in (no error)=w673) -> (error out=w667:errorcluster)  [unwired: 1 in, 2 out]
            n177 = Get Queue Status(queue=w669) -> (queue out=w668:refnum<queue>, error out=w666:errorcluster)  [unwired: 2 in, 6 out]
            n178 = case shown="No Error" w666 {
              tunnel: [w677 w679] -> w670
              tunnel: w668 -> [w676 _]
              tunnel: w667 -> [w675 w679]
              frame No Error {
                n179 = call "Enqueue Message (Single).vi"("error in (no error)"=w675, "Message"="Leave", "Message Queue"=w676) -> ("error out"=w677:errorcluster)  [unwired: 7 in, 1 out]
              }
              frame Error {
              }
            }
          }
          frame Default {
            n180 = xnode "Error Ring"("parameter 0"=w686) -> ("error out"=w687:errorcluster)
          }
        }
        n181 = call "Error Handler - Task Loop.vi"("error in (no error)"=w363, "Message Queue"=w367) -> ("dup error in"=w377:errorcluster)  [unwired: 8 in, 1 out]
        n182 = call <vilib>:"Clear Errors.vi"("error in (no error)"=w377) -> ("error out"=w350:errorcluster)  [unwired: 5 in, 1 out]
        "Loop-3 Iteration Counter 2" <- w364
      }
    }
    frame Enabled {
    }
  }
  n183 = case shown="No Error" "error in" {
    selector: "error in" -> [w700 w791]
    tunnel: [w699 w791] -> w2
    tunnel: "Message Queues" -> [w698 _]
    frame No Error {
      w693 = T4 {"Time (utc)"=0.0, "Data Out"=[]}  # Control Data
      w695 = T5 {"DAQ"={"ManagmentRate_Hz"=1, "StreamRate_Hz"=50, "StreamRate_ms"=20, "ManagmentRate_ms"=1000, "refDesArray"=[]}, "Modules"=[]}  # StreamCluster
      n184 = call <vilib>:"High Resolution Relative Seconds.vi"() -> ("relative seconds"=w694:dbl)
      n185 = Unbundle By Name(w698) -> ("UI"=w697:refnum<queue>, "Controls"=w696:refnum<queue>)
      n186 = while {
        shift-right: [w706] -> w699
        shift-left: w700 -> [w717]
        tunnel: w697 -> [w711]
        tunnel: w696 -> [w718]
        shift-right: [w705] -> _
        shift-left: w694 -> [w709]
        shift-right: [w703] -> _
        shift-left: w695 -> [w704]
        shift-right: [w702] -> _
        shift-left: w693 -> [w701]
        i -> [w708]
        stop <- w712 stop-if-true
        n187 = call <vilib>:"High Resolution Relative Seconds.vi"() -> ("relative seconds"=w705:dbl)
        n188 = Subtract(x=w705, y=w709) -> (x-y=→"Loop-3 Iteration Clock (s)":dbl)
        n189 = call "Dequeue Message.vi"("error in (no error)"=w717, "Message Queue"=w718) -> ("error out"=w716:errorcluster, "Message Data"=w714:variant, "Message"=w713:string, "dup Message Queue"=w715:refnum<queue>)  [unwired: 6 in]
        n190 = case shown="\"Start\"" w713 {
          selector: w713 -> [_ _ _ _ _ _ w784]
          tunnel: [w722 w726 w746 w758 w764 w773 w785] -> w707
          tunnel: w716 -> [w722 w727 w733 w759 w764 w775 _]
          tunnel: w715 -> [_ w728 w744 w757 _ w776 _]
          tunnel: w714 -> [_ _ _ _ w765 _ _]
          tunnel: [_ _ _ _ _ TRUE _] -> w712
          tunnel: w711 -> [_ _ _ _ _ w772 _]
          tunnel: w704 -> [w721 w725 w740 w756 w762 w768 w783]
          tunnel: [w720 w723 w737 w755 w760 w767 w782] -> w702
          tunnel: [w721 w725 w740 w756 w761 w768 w783] -> w703
          tunnel: w701 -> [w720 w723 w731 w755 w760 w767 w782]
          frame "Initialize" {
          }
          frame "Start" {
            n191 = call "Enqueue Message (Single).vi"("error in (no error)"=w727, "Message"="wsControl", "Message Queue"=w728) -> ("error out"=w726:errorcluster)  [unwired: 7 in, 1 out]
          }
          frame "wsControl" {
            n192 = Dequeue Element(queue="JSON cmd queue", timeout in ms (-1)=1, error in (no error)=w733) -> (element=w732:string, timed out?=w729:bool, error out=w730:errorcluster)  [unwired: 1 out]
            n193 = call "Enqueue Message (Single).vi"("error in (no error)"=w733, "Message"="wsControl", "Message Queue"=w744) -> ("error out"=w735:errorcluster)  [unwired: 7 in, 1 out]
            n194 = case shown="False" w729 {
              tunnel: [w747 w754] -> w739
              tunnel: w732 -> [_ w753]
              tunnel: w740 -> [_ w752]
              tunnel: w731 -> [w748 w751]
              tunnel: [w748 w750] -> w738
              tunnel: w730 -> [w747 w749]
              frame True {
              }
              frame False {
                n195 = call "cmdJsonToArrayId.vi"("error in"=w749, "Control Data"=w751, "StreamCluster"=w752, "JSON in"=w753) -> ("error out"=w754:errorcluster, "Control Data"=w750:T4)  [unwired: 6 in]
              }
            }
            n196 = call "doAoWrite.vi"("error in"=w739, "Control Data"=w738) -> ("error out"=w743:errorcluster, "Control Data"=w737:T4)  [unwired: 7 in, 1 out]
            n197 = Send Notification(notification=w737, notifier="Control Data Notifier", error in (no error)=w743) -> (error out=w736:errorcluster)  [unwired: 1 out]
            n198 = Merge Errors(w736, w735) -> (w746:errorcluster)
          }
          frame "Stop" {
            n199 = Flush Queue(queue=w757, error in (no error)=w759) -> (error out=w758:errorcluster)  [unwired: 2 out]
          }
          frame "Update Config" {
            n200 = Variant To Data(error in=w764, type=w762, Variant=w765) -> (data=w766:T5, error out=w763:errorcluster)
            n201 = Select(t=w762, s=w763, f=w766) -> (s? t:f=w761:T5)
          }
          frame "Leave" {
            n202 = Release Queue(queue=w776, error in (no error)=w775) -> (error out=w770:errorcluster)  [unwired: 1 in, 2 out]
            n203 = Get Queue Status(queue=w772) -> (queue out=w771:refnum<queue>, error out=w769:errorcluster)  [unwired: 2 in, 6 out]
            n204 = case shown="No Error" w769 {
              tunnel: [w779 w781] -> w773
              tunnel: w771 -> [w778 _]
              tunnel: w770 -> [w777 w781]
              frame No Error {
                n205 = call "Enqueue Message (Single).vi"("error in (no error)"=w777, "Message"="Leave", "Message Queue"=w778) -> ("error out"=w779:errorcluster)  [unwired: 7 in, 1 out]
              }
              frame Error {
              }
            }
          }
          frame Default {
            n206 = xnode "Error Ring"("parameter 0"=w784) -> ("error out"=w785:errorcluster)
          }
        }
        n207 = call "Error Handler - Task Loop.vi"("error in (no error)"=w707, "Message Queue"=w711) -> ("dup error in"=w719:errorcluster)  [unwired: 8 in, 1 out]
        n208 = call <vilib>:"Clear Errors.vi"("error in (no error)"=w719) -> ("error out"=w706:errorcluster)  [unwired: 5 in, 1 out]
        "Loop-3 Iteration Counter" <- w708
      }
    }
    frame Error {
    }
  }
  "error out" <- w2
